vi "Main_Host - Initialize Project Paths.vi"(8 "error in (no error)":errorcluster, 11 "Config Files Folder Path":path) -> (0 "error out":errorcluster, 3 "Config Files Folder Path":path)   [LabVIEW 2020]
doc: "JSMA Project Wizard 0.2.0.11\nRob Humfeld - JET Engineering\nCopyright (c) 2020, JET Engineering"
uses:
  Shared/Globals/Main_Host Config GBL.vi
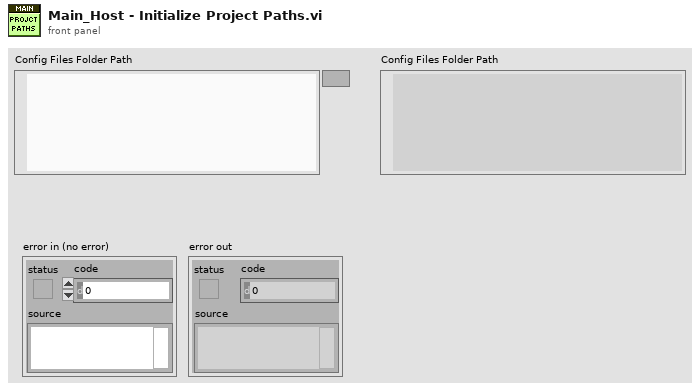
[diagram p1: front panel]
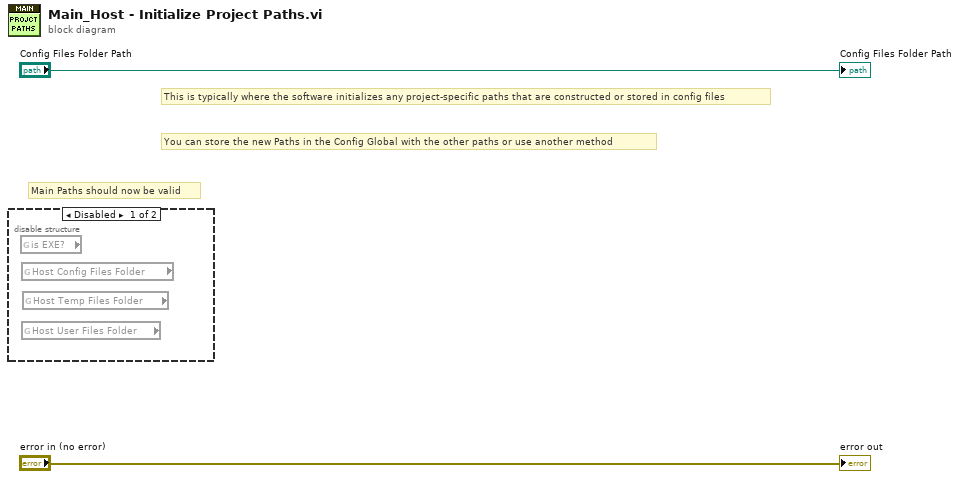
[diagram p0: block diagram]
diagram:
  # "Main Paths should now be valid"
  # "You can store the new Paths in the Config Global with the other paths or use another method"
  # "This is typically where the software initializes any project-specific paths that are constructed or stored in config files"
  n1 = disable-structure shown="Disabled" {
    frame Disabled {
      n2 = global read "Main_Host Config GBL.vi" "is EXE?"() -> ()  [unwired: 1 out]
      n3 = global read "Main_Host Config GBL.vi" "Host Config Files Folder"() -> ()  [unwired: 1 out]
      n4 = global read "Main_Host Config GBL.vi" "Host User Files Folder"() -> ()  [unwired: 1 out]
      n5 = global read "Main_Host Config GBL.vi" "Host Temp Files Folder"() -> ()  [unwired: 1 out]
    }
    frame Enabled {
    }
  }
  "error out" <- "error in (no error)"
  "Config Files Folder Path" <- "Config Files Folder Path"
